vi "FTW-URI-EscapeURL.vi"(0 "Input":string, 1 "Direction":enum16{"Encode", "Decode"}(ring)) -> (2 "Output":string)   [LabVIEW 2015]
panel:
  # "Inputs"
  # "Outputs"
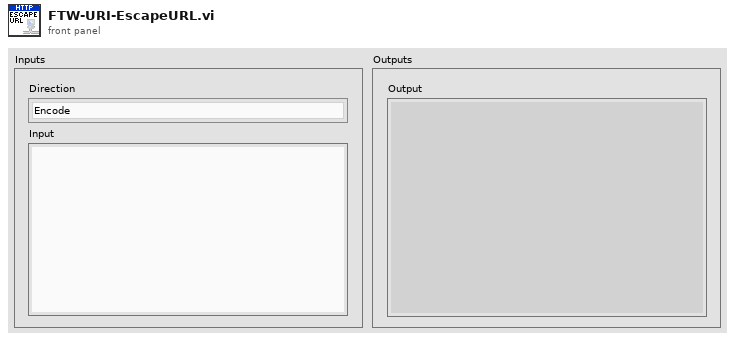
[diagram p1: front panel]
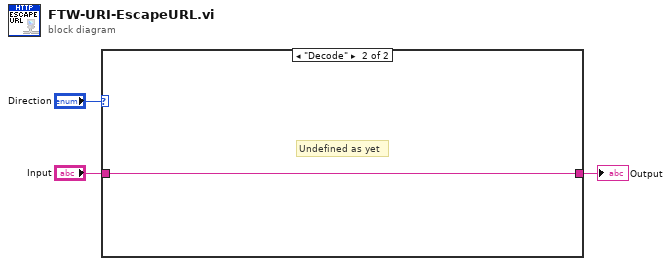
[diagram p0: block diagram]
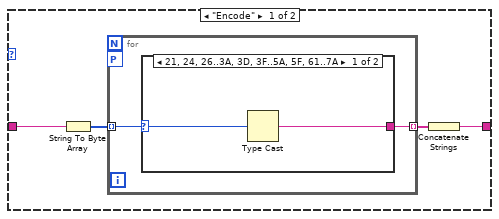
[diagram p2: hidden frame]
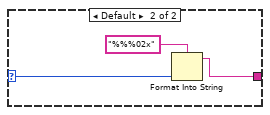
[diagram p3: hidden frame]
diagram:
  n1 = case shown="\"Decode\"" "Direction" {
    tunnel: [w6 w15] -> w1
    tunnel: "Input" -> [w7 w15]
    frame "Encode" {
      n2 = String To Byte Array(string=w7) -> (unsigned byte array=w5:u8[])
      n3 = for {
        tunnel: w5 -> [w9] mode=indexing
        tunnel: [w8] -> w4 mode=indexing
        workers-P: _ -> [_]
        n4 = case shown="21, 24, 26..3A, 3D, 3F..5A, 5F, 61..7A" w9 {
          selector: w9 -> [w11 w12]
          tunnel: [w10 w13] -> w8
          frame 33, 36, 38..58, 61, 63..90, 95, 97..122 {
            n5 = Type Cast(x=w11) -> (*(type *) &x=w10:string)  [unwired: 1 in]
          }
          frame Default {
            n6 = Format Into String(format string="%%%02x", w12) -> (resulting string=w13:string)  [unwired: 2 in, 1 out]
          }
        }
      }
      n7 = Concatenate Strings(w4) -> (w6:string)
    }
    frame "Decode" {
      # "Undefined as yet"
    }
  }
  "Output" <- w1
